vi "Image Aqq Close.vi"(1 "Error In":errorcluster, 3 "Session In":T1 caption="Camera") -> (0 "Error Out":errorcluster)   [LabVIEW 2015]
uses:
  <vilib>/userdefined/High Color/IMAQdx.ctl
  <vilib>/vision/driver/NI_Vision_Acquisition_Software.lvlib
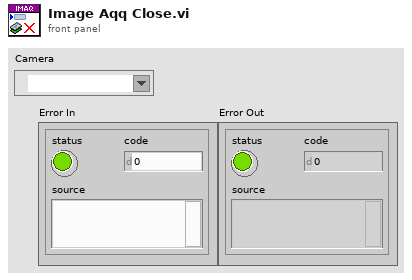
[diagram p1: front panel]
types:
  T1 = typedef "IMAQdx.ctl" = refnum<k21>
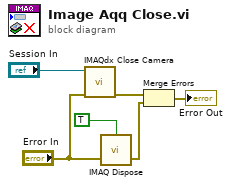
[diagram p0: block diagram]
diagram:
  n1 = call <vilib>:"IMAQdx Close Camera.vi"("error in"="Error In", "Session In"="Session In") -> ("error out"=w2:errorcluster)  [unwired: 9 in]
  n2 = call "IMAQ Dispose"("All Images? (No)"=TRUE, "error in (no error)"="Error In") -> ("error out"=w1:errorcluster)  [unwired: 4 in]
  n3 = Merge Errors(w2, w1) -> (→"Error Out":errorcluster)
